vi "LakeShore218_get_input_onoff.vi"(8 "error in":errorcluster, 10 "channel":i8=1, 11 "VISA in":refnum<visa-resource-name>) -> (0 "error out":errorcluster, 1 "onoff":enum16{"Off", "On"}(ring), 3 "VISA out":refnum<visa-resource-name>, 4 "status":bool)   [LabVIEW 2019]
panel:
  out "string":string
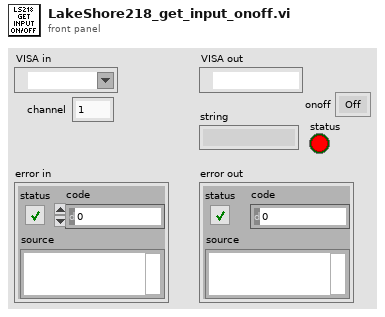
[diagram p1: front panel]
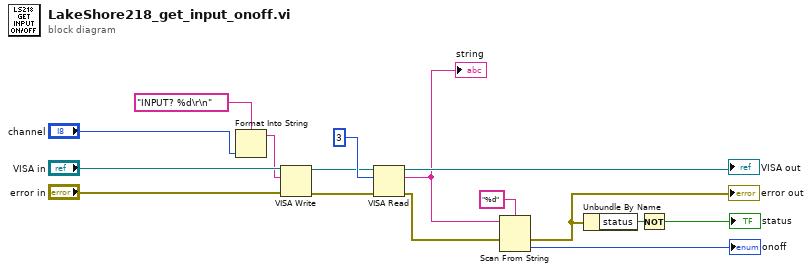
[diagram p0: block diagram]
diagram:
  n1 = Format Into String(format string="INPUT? %d\r\n", "channel") -> (resulting string=w3:string)  [unwired: 2 in, 1 out]
  n2 = VISA Write(VISA resource name="VISA in", write buffer=w3, error in (no error)="error in") -> (VISA resource name out=w4:refnum<visa-resource-name>, error out=w5:errorcluster)  [unwired: 1 out]
  n3 = VISA Read(VISA resource name=w4, byte count=u32 3, error in (no error)=w5) -> (VISA resource name out=→"VISA out":refnum<visa-resource-name>, read buffer=w12:string, error out=w10:errorcluster)  [unwired: 1 out]
  "string" <- w12
  n4 = Scan From String(format string="%d", input string=w12, error in=w10) -> (error out=w9:errorcluster, output 1=→"onoff":enum16{"Off", "On"})  [unwired: 2 in, 2 out]
  "error out" <- w9
  n5 = Unbundle By Name(w9) -> ("status"=w8:bool)
  n6 = Not(x=w8) -> (.not. x?=→"status":bool)
